vi "ReadData.vi"(8 "error in (no error)":errorcluster, 11 "NI_DAQmx(Angular) in":refnum<class "NI_DAQmx(Angular).lvclass">) -> (0 "error out":errorcluster, 2 "Waveform":waveform(dbl)[](array[waveform]), 3 "NI_DAQmx(Angular) out":refnum<class "NI_DAQmx(Angular).lvclass">)   [LabVIEW 2025, in "NI_DAQmx(Angular).lvclass"]
uses:
  NI_DAQmx(Angular).lvclass
  D:/Hardware/DAQ/DAQ_Abstr/Task_Abstr/Task_Abstr/Task_Abstr.lvclass
  D:/Hardware/DAQ/DAQ_Abstr/Task_Type/Waveform_Task/Waveform_Task/Waveform_Task.lvclass
  NI_DAQmx(Angular).lvclass/NI_DAQmx(Angular).ctl
  <vilib>/DAQmx/read.llb/DAQmx Read (Counter 2D DBL NChan NSamp).vi
  Read task.vi
  <vilib>/DAQmx/miscellaneous.llb/DAQmx Fill In Error Info.vi
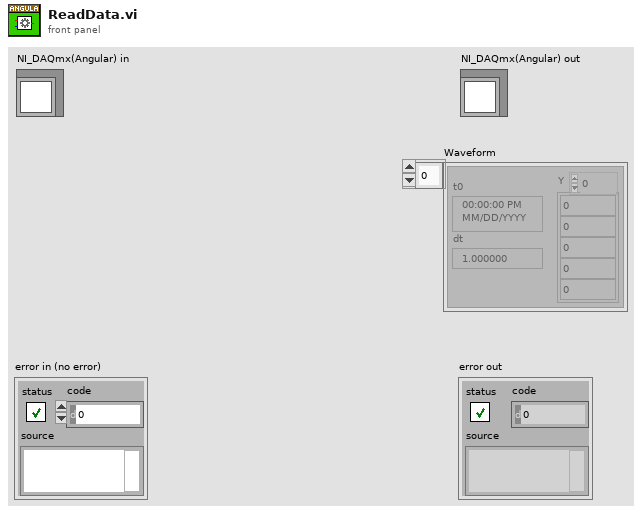
[diagram p1: front panel]
types:
  T1 = typedef "DAQ_Module.lvlib/DAQ_Module.lvclass/DAQ_Task_Config.ctl" = cluster{"Drive":T2, "TaskType":T3, "PhysicalChannels":string, "SampleRateConfiguration":T4, "ChannelConfig":map{string, cluster{"PhysicalChannels":string, "Config":string}}, "Enable":bool, "ShowPanel":bool}
  T2 = typedef "DAQ_Module.lvlib/DAQ_Module.lvclass/DAQ_HW_Type.ctl" = enum16{"NI_DAQmx", "Simulated_DAQ"}
  T3 = typedef "DAQ_Module.lvlib/DAQ_Module.lvclass/DAQ_Task_Type.ctl" = enum16{"AI", "Linear", "Angular", "AO"}
  T4 = typedef "DAQ_Module.lvlib/DAQ_Module.lvclass/DAQ_SampleRateConfig.ctl" = cluster{"SampleRate":dbl, "SamplesPerChannel":u32, "SamplesPerRead":i32, "SampleMode":i32, "Clock Source":string}
  T5 = map{string, cluster{"PhysicalChannels":string, "Config":string}}
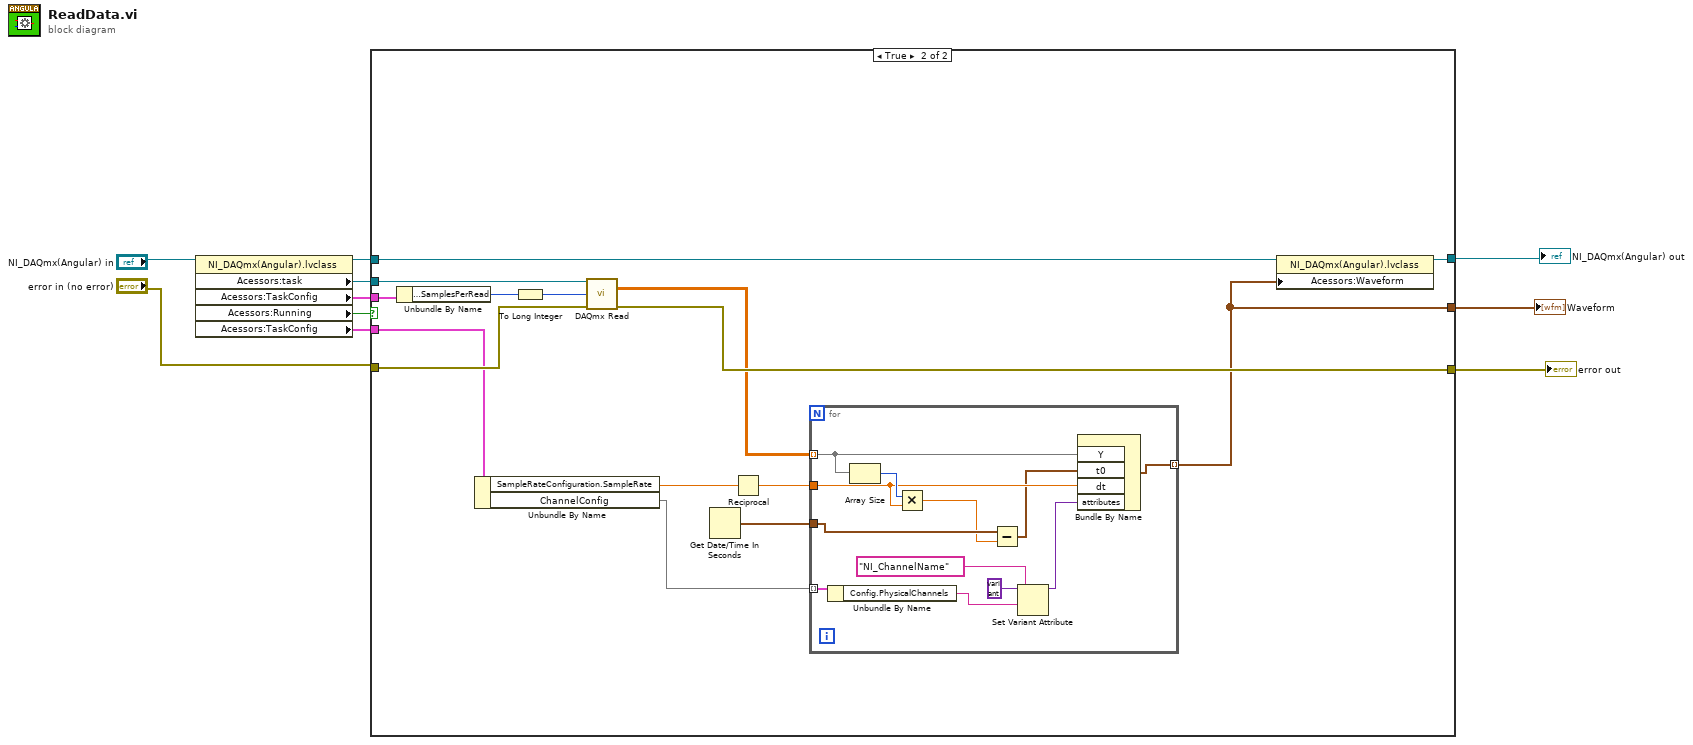
[diagram p0: block diagram]
diagram:
  n1 = property class="NI_DAQmx(Angular).lvclass"(reference="NI_DAQmx(Angular) in") -> (reference out=w8:refnum<class "NI_DAQmx(Angular).lvclass">, "Acessors:task"=w10:refnum<k21>, "Acessors:TaskConfig"=w9:T1, "Acessors:Running"=w7:bool, "Acessors:TaskConfig"=w6:T1)  [unwired: 1 in, 1 out]
  n2 = case shown="True" w7 {
    tunnel: w10 -> [_ w27]
    tunnel: "error in (no error)" -> [w11 w26]
    tunnel: [w11 w25] -> w2
    tunnel: w9 -> [_ w24]
    tunnel: w8 -> [w12 w21]
    tunnel: [w12 w20] -> w3
    tunnel: [_ w18] -> w1
    tunnel: w6 -> [_ w17]
    frame False {
    }
    frame True {
      n3 = Unbundle By Name(w24) -> ("SampleRateConfiguration.SamplesPerRead"=w23:i32)
      n4 = Unbundle By Name(w17) -> ("SampleRateConfiguration.SampleRate"=w16:dbl, "ChannelConfig"=w13:T5)
      n5 = To Long Integer(number=w23) -> (32bit integer=w22:i32)
      n6 = call-poly <vilib>:"DAQmx Read.vi"("task/channels in"=w27, "number of samples per channel"=w22, "error in"=w26) -> ("data"=w19:dbl[][], "error out"=w25:errorcluster)  [unwired: 10 in, 1 out]
      n7 = Get Date/Time In Seconds() -> (seconds since 1Jan1904=w14:timestamp)
      n8 = Reciprocal(x=w16) -> (1/x=w15:dbl)
      n9 = for {
        tunnel: w19 -> [w37] mode=indexing
        tunnel: [w39] -> w18 mode=indexing
        tunnel: w15 -> [w35]
        tunnel: w14 -> [w38]
        tunnel: w13 -> [w32] mode=indexing
        n10 = Unbundle By Name(w32) -> ("Config.PhysicalChannels"=w28:string)
        n11 = Array Size(array=w37) -> (size(s)=w36:i32)
        n12 = Multiply(x=w36, y=w35) -> (x*y=w34:dbl)
        n13 = Subtract(x=w38, y=w34) -> (x-y=w33:timestamp)
        n14 = Set Variant Attribute(Variant=variant ("variant"), name="NI_ChannelName", value=w28) -> (Variant out=w30:variant)  [unwired: 1 in, 2 out]
        n15 = Bundle By Name("Y"=w37, "t0"=w33, "dt"=w35, "attributes"=w30) -> (w39:waveform(dbl))  [unwired: 1 in]
      }
      n16 = property class="NI_DAQmx(Angular).lvclass"(reference=w21, "Acessors:Waveform"=w18) -> (reference out=w20:refnum<class "NI_DAQmx(Angular).lvclass">)  [unwired: 1 in, 1 out]
    }
  }
  "error out" <- w2
  "NI_DAQmx(Angular) out" <- w3
  "Waveform" <- w1
